vi "get result path start.vi"(0 "main VI path":path) -> (4 "result file path":path)   [LabVIEW 2019]
doc: "This subVI uses the main VI's path as a reference pointer to choose the result data file path."
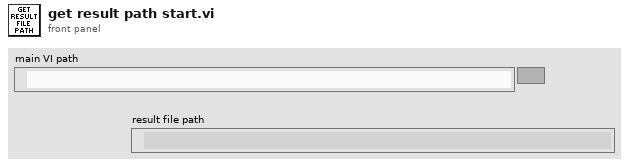
[diagram p1: front panel]
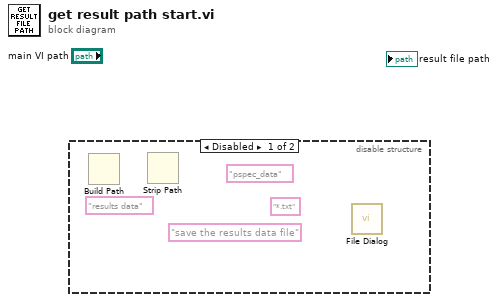
[diagram p0: block diagram]
diagram:
  n1 = disable-structure shown="Disabled" {
    frame Disabled {
      (unwired) "results data" ("name or relative path")
      (unwired) "save the results data file" ("prompt")
      (unwired) "pspec_data" ("default name")
      (unwired) "*.txt" ("pattern (all files)")
      n2 = Build Path() -> ()  [unwired: 2 in, 1 out]
      n3 = Strip Path() -> ()  [unwired: 1 in, 2 out]
      n4 = call "File Dialog"() -> ()  [unwired: 12 in, 4 out]
    }
    frame Enabled {
    }
  }
